vi "Wait until SPI is Idle.vi"(7 "Timeout (s)":dbl=5.0 caption="Time Target (s)", 8 "error in":errorcluster, 11 "FPGA VI Reference In":refnum<k20>) -> (0 "error out":errorcluster, 2 "SPI Idle?":bool=TRUE, 3 "FPGA VI Reference Out":refnum<k20>)   [LabVIEW 2012]
doc: "This VI initializes adpater mddule"
uses:
  <vilib>/rvi/errors/niLvFpgaAdjustHostInterfaceError.vi
  <vilib>/rvi/interface/nirviReadWriteControl/nirviReadWriteControl.xnode
  NiFpgaLv.dll
  <vilib>/rvi/interface/Simulation/niFpgaSimulationCallBeginRW.vi
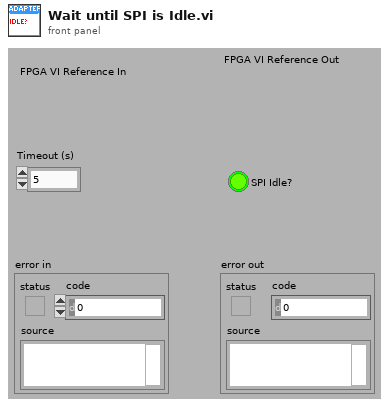
[diagram p1: front panel]
types:
  T1 = cluster{"io mod.initialization done":bool, "io mod.configuration error":bool, "io mod.synthesizer locked":bool, "io mod.spi idle":bool}
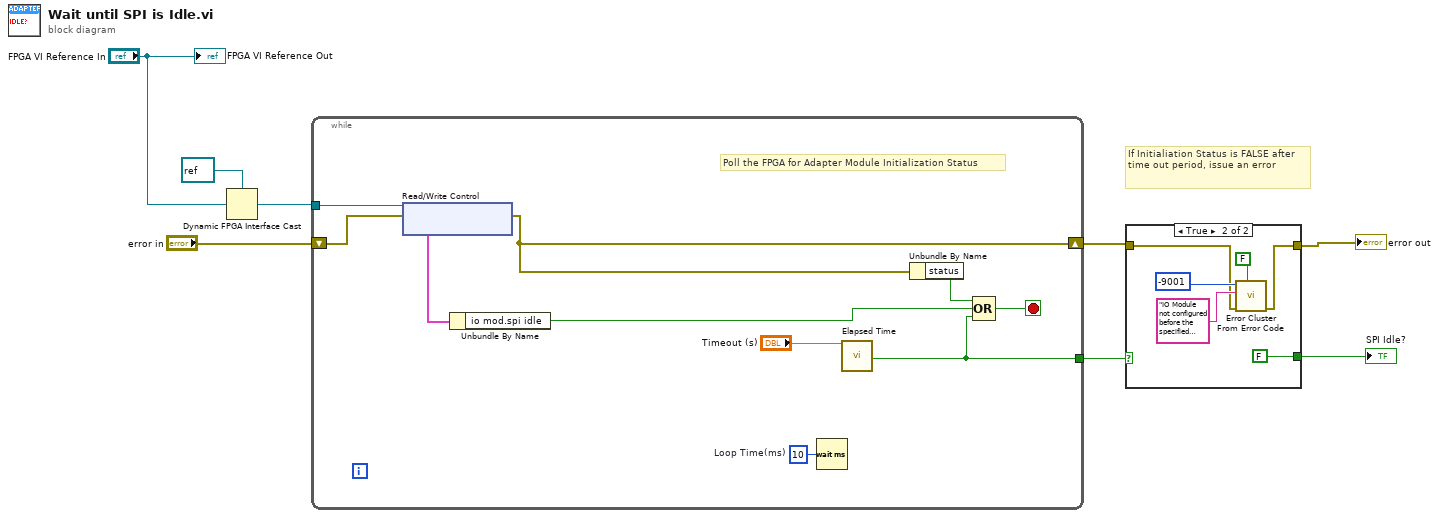
[diagram p0: block diagram]
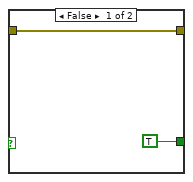
[diagram p2: hidden frame]
diagram:
  # "If Initialiation Status is FALSE after time out period, issue an error"
  n1 = Dynamic FPGA Interface Cast(Session In=refnum<k20> refnum ("Type"), Type="FPGA VI Reference In") -> (Session Out=w3:refnum<k20>)
  n2 = while {
    shift-right: [w10] -> w7
    shift-left: "error in" -> [w12]
    tunnel: [w14] -> w6
    tunnel: w3 -> [w13]
    stop <- w17 stop-if-true
    w18 = u32 10  # Loop Time(ms)
    # "Poll the FPGA for Adapter Module Initialization Status"
    n3 = xnode "Read/Write Control"("FPGA VI Reference In"=w13, "error in"=w12) -> ("error out"=w10:errorcluster, "IO Module Status"=w11:T1)  [unwired: 1 out]
    n4 = Unbundle By Name(w11) -> ("io mod.spi idle"=w9:bool)
    n5 = Wait (ms)(milliseconds to wait=w18) -> ()  [unwired: 1 out]
    n6 = call "Elapsed Time"("Time Target (s)"="Timeout (s)") -> ("Time has Elapsed"=w14:bool)  [unwired: 11 in, 7 out]
    n7 = Unbundle By Name(w10) -> ("status"=w16:bool)
    n8 = Compound Arithmetic op=OR(w16, w9, w14) -> (w17:bool)
  }
  n9 = case shown="True" w6 {
    tunnel: w7 -> [w20 w22]
    tunnel: [w20 w25] -> w5
    tunnel: [TRUE ("Master FAM Configured") FALSE ("Master FAM Configured")] -> w4
    frame False {
    }
    frame True {
      n10 = call <vilib>:"Error Cluster From Error Code.vi"("show call chain? (False)"=FALSE, "error in (no error)"=w22, "error message (\"\")"="IO Module not configured before the specified timeout." ("source"), "error code (0)"=-9001 ("code")) -> ("error out"=w25:errorcluster)  [unwired: 5 in]
    }
  }
  "error out" <- w5
  "SPI Idle?" <- w4
  "FPGA VI Reference Out" <- "FPGA VI Reference In"
